vi "Empty RX buffer.vi"(8 "error in (no error)":errorcluster, 11 "RP Instrument in":refnum<class "RP Instrument.lvclass">) -> (0 "error out":errorcluster, 2 "Data out":i32[](array[numeric]), 3 "RP Instrument out":refnum<class "RP Instrument.lvclass">)   [LabVIEW 2015, in "RP Instrument.lvclass"]
uses:
  RP Instrument.lvclass
  RP Instrument.lvclass/RP Instrument.ctl
  RP Communicator/RP Communicator.lvclass
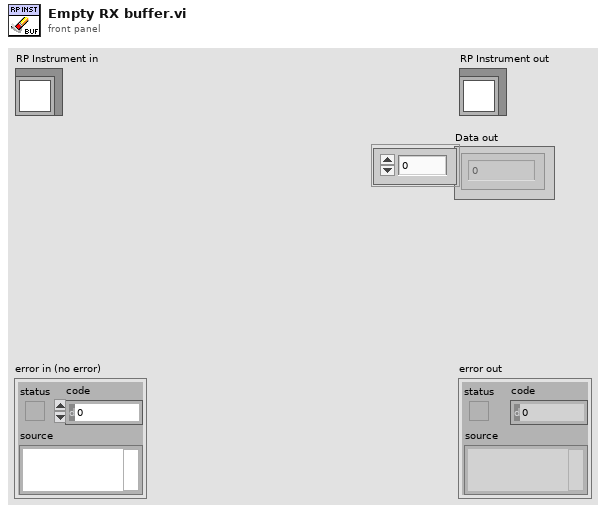
[diagram p1: front panel]
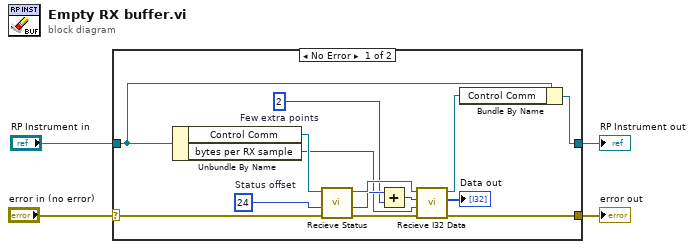
[diagram p0: block diagram]
diagram:
  n1 = case shown="No Error" "error in (no error)" {
    selector: "error in (no error)" -> [w12 w20]
    tunnel: [w11 w20] -> w3
    tunnel: [w17 w19] -> w1
    tunnel: "RP Instrument in" -> [w18 w19]
    frame No Error {
      w6 = u32 2  # Few extra points
      w16 = u64 24  # Status offset
      n2 = Unbundle By Name(w18) -> ("Control Comm"=w15:refnum<class "RP Communicator.lvclass">, "bytes per RX sample"=w5:u32)
      n3 = call-dynamic "Recieve Status.vi"("error in (no error)"=w12, "Status offset"=w16, "RP Communicator in"=w15) -> ("error out"=w13:errorcluster, "Status response"=w7:u32, "RP Communicator out"=w14:refnum<class "RP Communicator.lvclass">)  [unwired: 6 in]
      n4 = Add(x=w7, y=w6) -> (x+y=w8:u32)
      n5 = call-dynamic "Recieve I32 Data.vi"("error in (no error)"=w13, "bytes per sample"=w5, "Samples per read"=w8, "RP Communicator in"=w14) -> ("error out"=w11:errorcluster, "Data out"=→"Data out":i32[], "RP Communicator out"=w9:refnum<class "RP Communicator.lvclass">)  [unwired: 5 in]
      n6 = Bundle By Name(cluster=w18, "Control Comm"=w9) -> (w17:refnum<class "RP Instrument.lvclass">)
    }
    frame Error {
    }
  }
  "error out" <- w3
  "RP Instrument out" <- w1
